vi "S_to_Y.vi"(2 "error in (no error)":errorcluster, 3 "Reference Impedance":dbl=50.0, 4 "Input S-parameter Trace Array":T2(array[cluster]) {"Freq (Hz)" format="%.2e"; "S-parameter Array" format="%.2f"}) -> (0 "error out":errorcluster, 1 "Output Y-parameter Trace Array":T1(array[cluster]) {"Freq (Hz)" format="%.2e"; "Y-parameter Array" format="%.2f"})   [LabVIEW 2017]
uses:
  <vilib>/Analysis/baseanly.llb/Complex A x B.vi
  <vilib>/Analysis/baseanly.llb/Complex Inverse Matrix.vi
  <vilib>/Analysis/Matrix/Numeric/Multiply/Multiply - C,CM.vi
  <vilib>/Analysis/NI_AALBase.lvlib
  <vilib>/Analysis/Matrix/NI_Matrix.lvlib
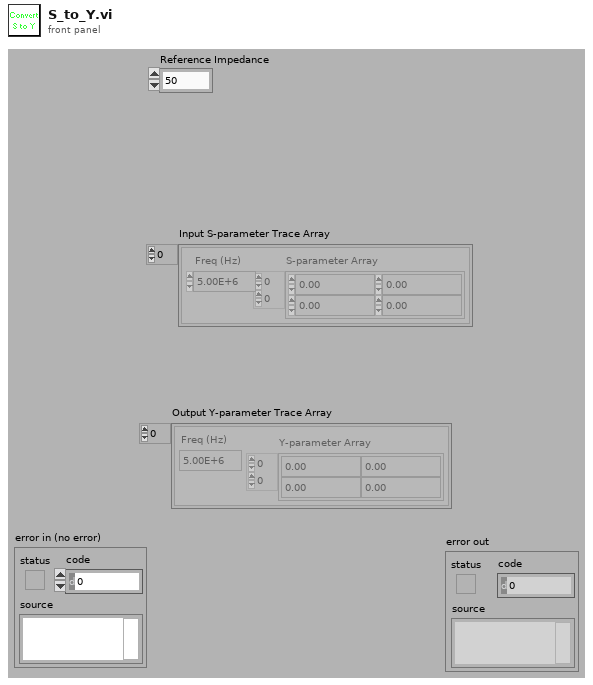
[diagram p1: front panel]
types:
  T1 = cluster{"Freq (Hz)":dbl, "Y-parameter Array":csg[][]}[]
  T2 = cluster{"Freq (Hz)":dbl, "S-parameter Array":csg[][]}[]
  T3 = typedef "NI_Matrix.lvlib/ComplexMatrix.ctl" = cdb[][]
  T4 = cluster{"Freq (Hz)":dbl, "Y-parameter Array":csg[][]}
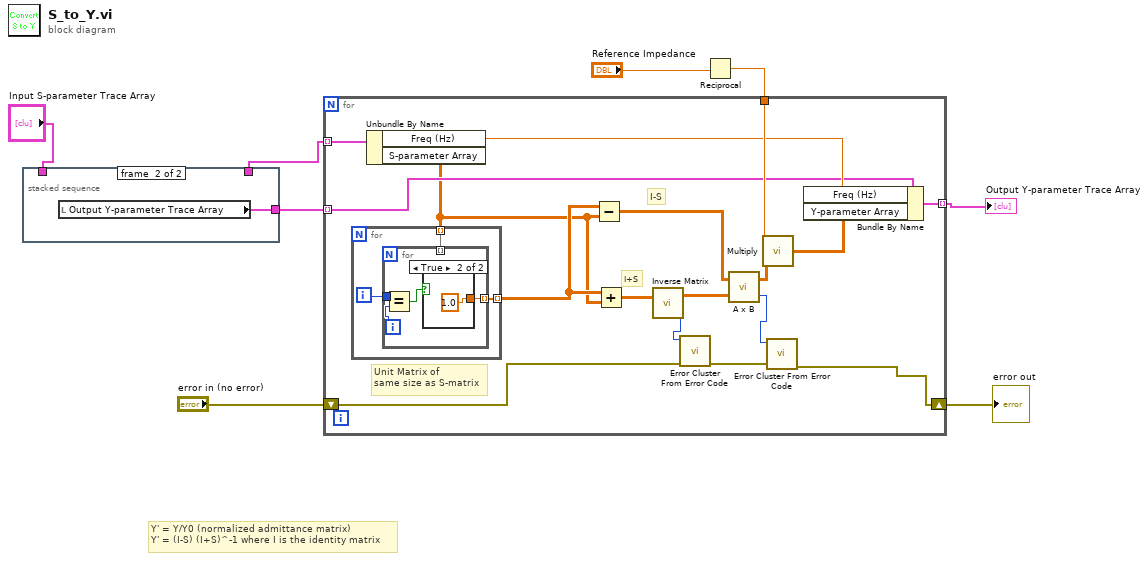
[diagram p0: block diagram]
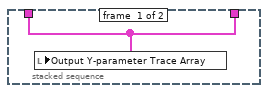
[diagram p2: hidden frame]
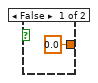
[diagram p3: hidden frame]
diagram:
  # "Y' = Y/Y0 (normalized admittance matrix)\nY' = (I-S) (I+S)^-1 where I is the identity matrix"
  n1 = stacked-sequence {
    tunnel: "Input S-parameter Trace Array" -> [w9 _]
    tunnel: [w9 _] -> w2
    tunnel: [_ w10] -> w1
    frame #0 {
      n2 = local write "Output Y-parameter Trace Array"(w9) -> ()
    }
    frame #1 {
      n3 = local read "Output Y-parameter Trace Array"() -> (w10:T1)
    }
  }
  n4 = Reciprocal(x="Reference Impedance") -> (1/x=w7:dbl)
  n5 = for {
    tunnel: w2 -> [w27] mode=indexing
    tunnel: w7 -> [w23]
    tunnel: [w19] -> w6 mode=indexing
    shift-right: [w14] -> w4
    shift-left: "error in (no error)" -> [w16]
    tunnel: w1 -> [w13] mode=indexing
    # "I+S"
    # "I-S"
    # "Unit Matrix of\nsame size as S-matrix"
    n6 = Unbundle By Name(w27) -> ("Freq (Hz)"=w21:dbl, "S-parameter Array"=w11:csg[][])
    n7 = for {
      tunnel: w11 -> [w30] mode=indexing
      tunnel: [w28] -> w12 mode=indexing
      i -> [w29]
      n8 = for {
        tunnel: w30 -> [_] mode=indexing
        tunnel: w29 -> [w33]
        tunnel: [w31] -> w28 mode=indexing
        i -> [w34]
        n9 = Equal?(x=w33, y=w34) -> (x = y?=w32:bool)
        n10 = case shown="True" w32 {
          tunnel: [0.0 1.0] -> w31
          frame False {
          }
          frame True {
          }
        }
      }
    }
    n11 = Subtract(x=w12, y=w11) -> (x-y=w25:cdb[][])
    n12 = Add(x=w12, y=w11) -> (x+y=w26:cdb[][])
    n13 = call-poly <vilib>:"Inverse Matrix.vi"("Input Matrix"=w26) -> ("error"=w18:i32, "Inverse Matrix"=w24:T3)  [unwired: 1 in]
    n14 = call <vilib>:"Error Cluster From Error Code.vi"("error in (no error)"=w16, "error code (0)"=w18) -> ("error out"=w15:errorcluster)  [unwired: 1 in, 6 out]
    n15 = call-poly <vilib>:"A x B.vi"("B"=w24, "A"=w25) -> ("error"=w17:i32, "A x B"=w22:T3)
    n16 = call-poly <vilib>:"Multiply.vi"("Complex Matrix A"=w22, "Complex Scalar c"=w23) -> ("c * A"=w20:T3)
    n17 = call <vilib>:"Error Cluster From Error Code.vi"("error in (no error)"=w15, "error code (0)"=w17) -> ("error out"=w14:errorcluster)  [unwired: 1 in, 6 out]
    n18 = Bundle By Name(cluster=w13, "Freq (Hz)"=w21, "Y-parameter Array"=w20) -> (w19:T4)
  }
  "Output Y-parameter Trace Array" <- w6
  "error out" <- w4
